vi "Get Users.vi"(8 "error in (no error)":errorcluster, 11 "Data.PG":refnum<class "LV-Data.PGSQL.lvclass">) -> (0 "error out":errorcluster, 2 "Users":string[](array[string]), 3 "Data.PG out":refnum<class "LV-Data.PGSQL.lvclass">)   [LabVIEW 2019, in "LV-Data.PGSQL.lvclass"]
uses:
  LV-Data.PGSQL.lvclass
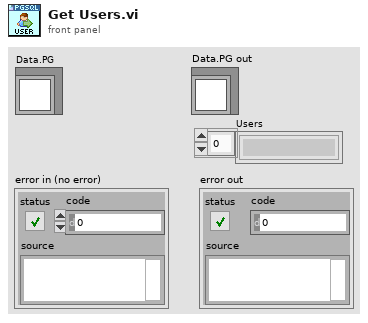
[diagram p1: front panel]
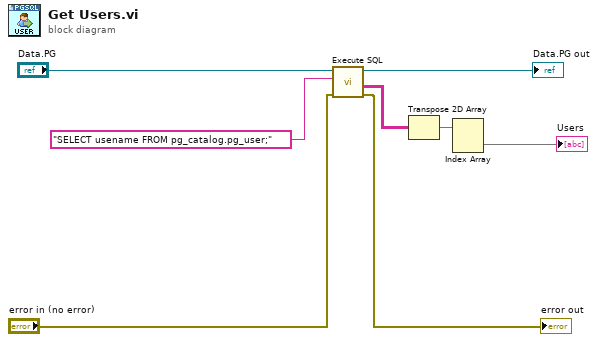
[diagram p0: block diagram]
diagram:
  n1 = call "Execute SQL.vi"("error in"="error in (no error)", "SQL"="SELECT usename FROM pg_catalog.pg_user;" ("command"), "LV-Data.PGSQL"="Data.PG") -> ("error out"=→"error out":errorcluster, "Result"=w1:string[][], "LV-Data.PGSQL out"=→"Data.PG out":refnum<class "LV-Data.PGSQL.lvclass">)  [unwired: 5 in, 1 out]
  n2 = Transpose 2D Array(2D array=w1) -> (transposed array=w5:string[][])
  n3 = Index Array(array=w5) -> (element=→"Users":string[])  [unwired: 2 in]
